vi "switching_test.vi"() -> ()   [LabVIEW 2020]
uses:
  Realization/PIPX40 Relay/PIPX40 Relay.lvclass
panel:
  in  "List":i32[](array[numeric])
  out "Boolean array":bool[][](array[boolean])
  out "error out":errorcluster
  out "pattern":u32[](array[numeric])
  in  "Relay":refnum<visa-resource-name>="PXI14::11::INSTR"
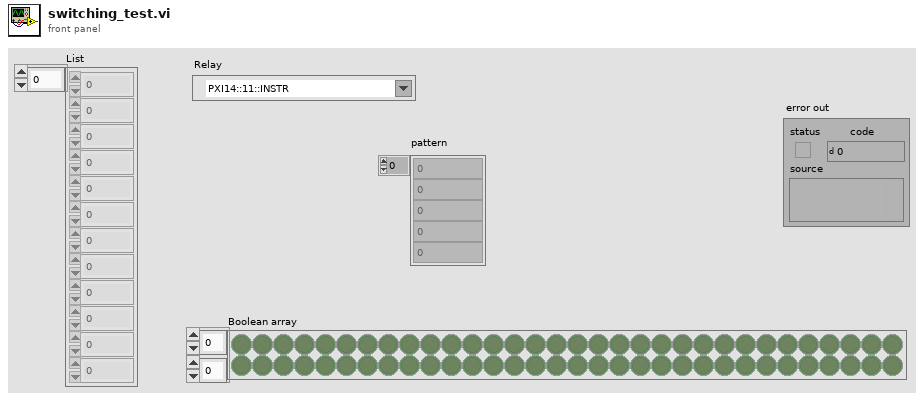
[diagram p1: front panel]
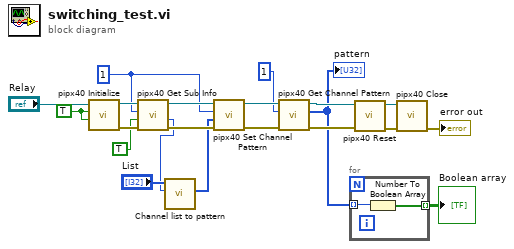
[diagram p0: block diagram]
diagram:
  w3 = u32 1 ("subunit number")
  w20 = TRUE ("id query")
  n1 = call <instrlib>:"pipx40 Initialize.vi"("reset device"=w20, "id query"=w20, "resource name"="Relay") -> ("error out"=w7:errorcluster, "instrument handle out"=w8:refnum<visa-resource-name>)  [unwired: 7 in]
  n2 = call <instrlib>:"pipx40 Get Sub Info.vi"("error in (no error)"=w7, "is output"=TRUE, "subunit number"=w3, "instrument handle"=w8) -> ("error out"=w5:errorcluster, "columns"=w1:u32, "instrument handle out"=w4:refnum<visa-resource-name>)  [unwired: 3 in, 2 out]
  n3 = call "Channel list to pattern.vi"("Outputs"=w1, "List"="List") -> ("Pattern"=w2:u32[])  [unwired: 9 in]
  n4 = call <instrlib>:"pipx40 Set Channel Pattern.vi"("error in (no error)"=w5, "pattern"=w2, "subunit number"=w3, "instrument handle"=w4) -> ("error out"=w16:errorcluster, "instrument handle out"=w17:refnum<visa-resource-name>)  [unwired: 6 in]
  n5 = call <instrlib>:"pipx40 Get Channel Pattern.vi"("error in (no error)"=w16, "subunit number"=u32 1, "instrument handle"=w17) -> ("error out"=w15:errorcluster, "pattern"=w11:u32[], "instrument handle out"=w14:refnum<visa-resource-name>)  [unwired: 6 in]
  "pattern" <- w11
  n6 = for {
    tunnel: w11 -> [w23] mode=indexing
    tunnel: [w22] -> w10 mode=indexing
    n7 = Number To Boolean Array(number=w23) -> (Boolean array=w22:bool[])
  }
  "Boolean array" <- w10
  n8 = call <instrlib>:"pipx40 Reset.vi"("error in (no error)"=w15, "instrument handle"=w14) -> ("error out"=w19:errorcluster, "instrument handle out"=w18:refnum<visa-resource-name>)  [unwired: 8 in]
  n9 = call <instrlib>:"pipx40 Close.vi"("error in (no error)"=w19, "instrument handle"=w18) -> ("error out"=→"error out":errorcluster)  [unwired: 9 in]
